vi "UpdateText.vi"(8 "ErrorIn":errorcluster, 9 "ID":string, 10 "JSONText":string, 11 "ReferenceIn":refnum<class "JSONTextViewer.lvclass">) -> (0 "ErrorOut":errorcluster, 3 "ReferenceOut":refnum<class "JSONTextViewer.lvclass">)   [LabVIEW 2021, in "JSONTextViewer.lvlib" / "JSONTextViewer.lvclass"]
uses:
  JSONTextViewer.lvclass
  6ddda736-cc5f-4252-898b-cf7bf48c6d8e.vi
  protected/MainGUIRepository.vi
  JSONTextViewer.lvclass/JSONTextViewer.ctl
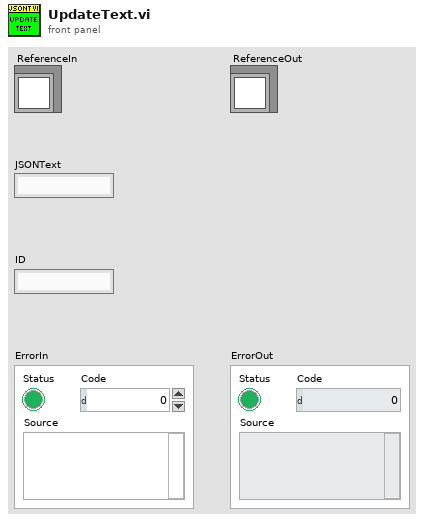
[diagram p1: front panel]
types:
  T1 = typedef "JSONTextViewer.lvlib/JSONTextViewer.lvclass/ObjectAttributes.ctl" = cluster{"Interfaces":cluster{"ApplicationConfiguration":refnum<class "IApplicationConfiguration.lvclass">}, "Locals":cluster{"MainGUIActive":refnum<queue>, "JSONText":string, "ID":string}, "Persistent":cluster{"Dummy":bool}}
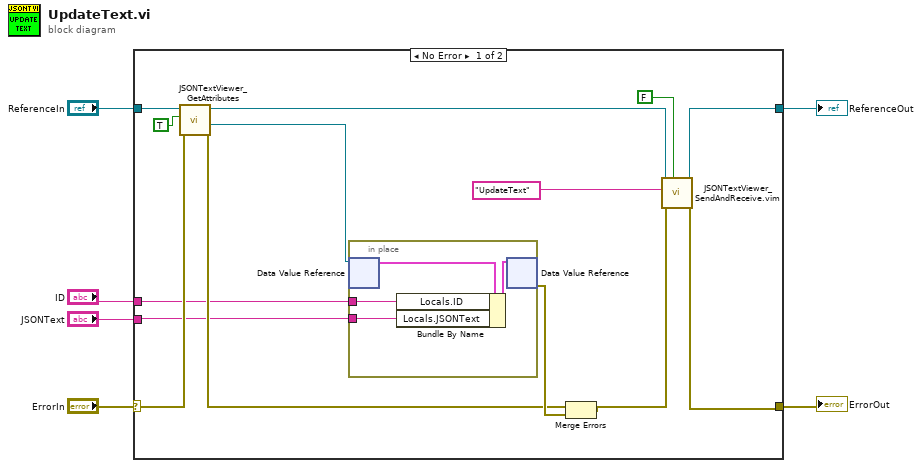
[diagram p0: block diagram]
diagram:
  n1 = case shown="No Error" "ErrorIn" {
    selector: "ErrorIn" -> [w19 w26]
    tunnel: [w16 w26] -> w5
    tunnel: [w10 w25] -> w3
    tunnel: "ReferenceIn" -> [w15 w25]
    tunnel: "JSONText" -> [w12 _]
    tunnel: "ID" -> [w7 _]
    frame No Error {
      n2 = call "JSONTextViewer_GetAttributes.vi"("ErrorIn"=w19, "OnlyGetDvrReference(False)"=TRUE, "ReferenceIn"=w15) -> ("ErrorOut"=w18:errorcluster, "DataRef"=w13:refnum<data-value>, "ReferenceOut"=w11:refnum<class "JSONTextViewer.lvclass">)  [unwired: 5 in, 1 out]
      n3 = in-place {
        in-place-border: w12 -> [w22]
        in-place-border: w7 -> [w21]
        n4 = in-place-dvr #1(w13) -> (w24:T1)  [unwired: 1 out]
        n5 = Bundle By Name(cluster=w24, "Locals.ID"=w21, "Locals.JSONText"=w22) -> (w23:T1)
        n6 = in-place-dvr #1(w23) -> (w20:errorcluster)  [unwired: 1 out]
      }
      n7 = Merge Errors(w18, w20) -> (w17:errorcluster)
      n8 = call "JSONTextViewer_SendAndReceive.vim"("ShouldWeWaitForResponse"=FALSE, "ErrorIn"=w17, "Command"="UpdateText", "ReferenceIn"=w11) -> ("ErrorOut"=w16:errorcluster, "ReferenceOut"=w10:refnum<class "JSONTextViewer.lvclass">)  [unwired: 5 in, 1 out]
    }
    frame Error {
    }
  }
  "ErrorOut" <- w5
  "ReferenceOut" <- w3
